vi "Initialize.vi"(8 "error in (no error)":errorcluster, 9 "Reset (True)":bool=TRUE, 10 "ID Query (True)":bool=TRUE, 11 "VISA resource name":refnum<visa-resource-name>) -> (0 "error out":errorcluster, 3 "VISA resource name out":refnum<visa-resource-name>)   [LabVIEW 2024, in "Agilent 532XX Series.lvlib"]
doc: "Establishes communication with the instrument and optionally performs an instrument identification query and/or an instrument reset. It also places the instrument in a default state needed for other instrument driver operations. Therefore, call this VI before calling other instrument driver VIs for this instrument. Generally, you need to call the Initialize VI only once at the beginning of an application."
uses:
  Agilent 532XX Series.lvlib
  <vilib>/regexp/Match Regular Expression.xnode
panel:
  # "(c) 2010-2015 National Instruments.  ALL RIGHTS RESERVED."
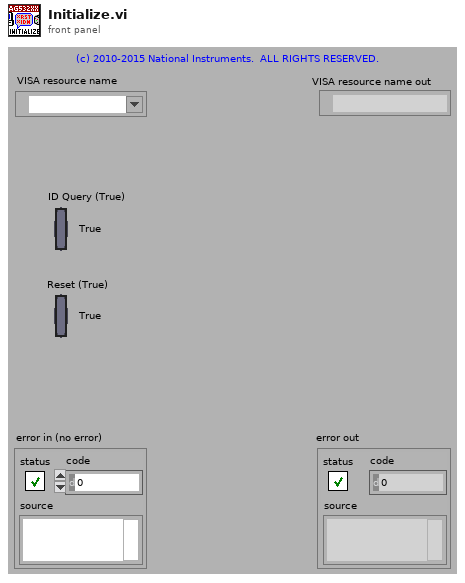
[diagram p1: front panel]
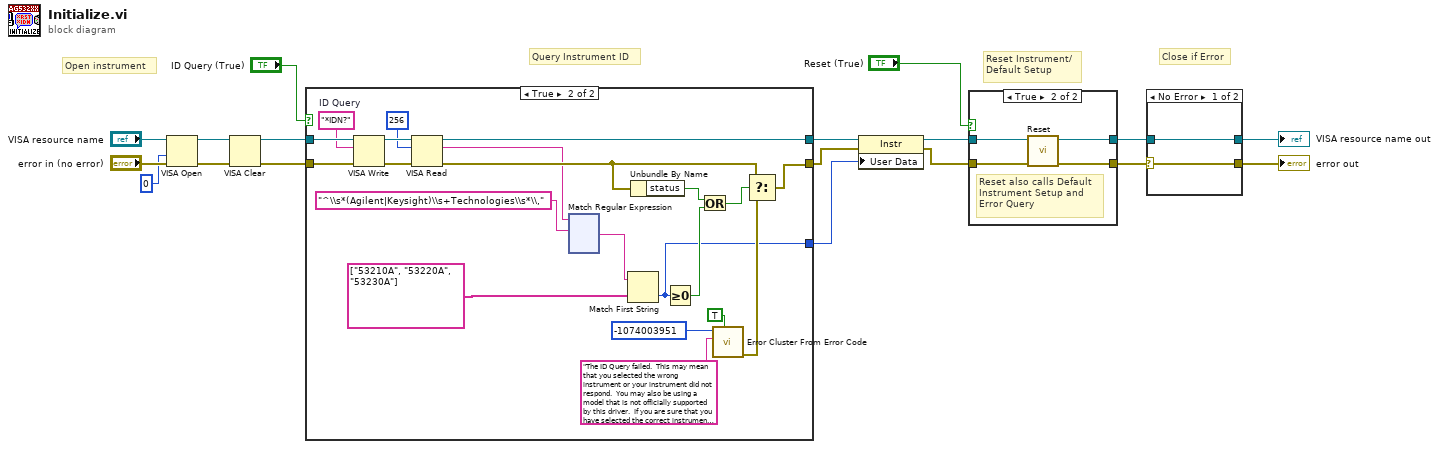
[diagram p0: block diagram]
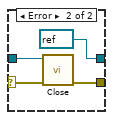
[diagram p2: hidden frame]
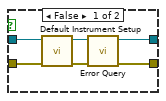
[diagram p3: hidden frame]
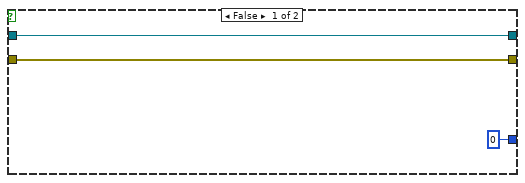
[diagram p4: hidden frame]
diagram:
  # "Close if Error"
  # "Query Instrument ID"
  # "Reset Instrument/\nDefault Setup"
  # "Open instrument"
  n1 = VISA Open(access mode=u32 0, error in (no error)="error in (no error)", VISA resource name="VISA resource name") -> (VISA resource name=w13:refnum<visa-resource-name>, error out=w12:errorcluster)  [unwired: 2 out]
  n2 = VISA Clear(VISA resource name=w13, error in (no error)=w12) -> (VISA resource name out=w7:refnum<visa-resource-name>, error out=w6:errorcluster)
  n3 = case shown="True" "ID Query (True)" {
    tunnel: [w20 w42] -> w4
    tunnel: [w21 w39] -> w5
    tunnel: w7 -> [w21 w40]
    tunnel: w6 -> [w20 w41]
    tunnel: [0 ("index") w25] -> w1
    frame False {
    }
    frame True {
      w35 = "*IDN?"  # ID Query
      n4 = VISA Write(VISA resource name=w40, write buffer=w35, error in (no error)=w41) -> (VISA resource name out=w38:refnum<visa-resource-name>, error out=w37:errorcluster)  [unwired: 1 out]
      n5 = VISA Read(VISA resource name=w38, byte count=u32 256, error in (no error)=w37) -> (VISA resource name out=w39:refnum<visa-resource-name>, read buffer=w22:string, error out=w30:errorcluster)  [unwired: 1 out]
      n6 = xnode ("Match Regular Expression")("input string"=w22, "regular expression"="^\\s*(Agilent|Keysight)\\s+Technologies\\s*\\," ("Company Name Regular Expression")) -> ("after match"=w23:string)  [unwired: 4 in, 4 out]
      n7 = Match First String(2:string[] ["53210A", "53220A", "53230A"], 3:w23) -> (0:w25:i32)  [unwired: 1 out]
      n8 = Unbundle By Name(w30) -> ("status"=w29:bool)
      n9 = Greater Or Equal To 0?(x=w25) -> (x >= 0?=w28:bool)
      n10 = Or(x=w29, y=w28) -> (x .or. y?=w27:bool)
      n11 = call <vilib>:"Error Cluster From Error Code.vi"("show call chain? (False)"=TRUE, "error message (\"\")"="The ID Query failed.  This may mean that you selected the wrong instrument or your instrument did not respond.  You may also be using a model that is not officially supported by this driver.  If you are sure that you have selected the correct instrument and it is responding, try disabling the ID Query." ("Source (VI Name)"), "error code (0)"=-1074003951 ("Code")) -> ("error out"=w34:errorcluster)  [unwired: 1 in, 5 out]
      n12 = Select(t=w30, s=w27, f=w34) -> (s? t:f=w42:errorcluster)
    }
  }
  n13 = property class="Instr"(reference=w5, error in=w4, "User Data"=w1) -> (reference out=w3:refnum<visa-resource-name>, error out=w2:errorcluster)
  n14 = case shown="True" "Reset (True)" {
    tunnel: w2 -> [w164 w166]
    tunnel: [w161 w169] -> w8
    tunnel: w3 -> [w165 w167]
    tunnel: [w162 w168] -> w9
    frame False {
      n15 = call "Default Instrument Setup.vi"("error in (no error)"=w164, "VISA resource name"=w165) -> ("error out"=w160:errorcluster, "VISA resource name out"=w163:refnum<visa-resource-name>)  [unwired: 8 out]
      n16 = call "Error Query.vi"("error in (no error)"=w160, "VISA resource name"=w163) -> ("error out"=w161:errorcluster, "VISA resource name out"=w162:refnum<visa-resource-name>)  [unwired: 8 out]
    }
    frame True {
      # "Reset also calls Default Instrument Setup and Error Query"
      n17 = call "Reset.vi"("error in (no error)"=w166, "VISA resource name"=w167) -> ("error out"=w169:errorcluster, "VISA resource name out"=w168:refnum<visa-resource-name>)  [unwired: 8 out]
    }
  }
  n18 = case shown="No Error" w8 {
    selector: w8 -> [w170 w173]
    tunnel: w9 -> [w171 w174]
    tunnel: [w171 refnum<visa-resource-name> refnum ("VISA resource name out")] -> w11
    tunnel: [w170 w175] -> w10
    frame No Error {
    }
    frame Error {
      n19 = call "Close.vi"("error in (no error)"=w173, "VISA resource name"=w174) -> ("error out"=w175:errorcluster)  [unwired: 9 out]
    }
  }
  "VISA resource name out" <- w11
  "error out" <- w10
